vi "Read_Sc.vi"(3 "error in (no error)":errorcluster, 4 "timeout ms (10000)":i32=10000, 5 "connection ID":refnum<k5>) -> (0 "error out":errorcluster, 1 "data out":string, 2 "connection ID out":refnum<k5>)   [LabVIEW 2015]
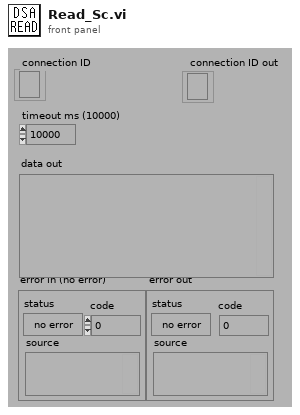
[diagram p1: front panel]
types:
  T1 = enum16{"Standard", "Buffered", "CRLF", "Immediate"}
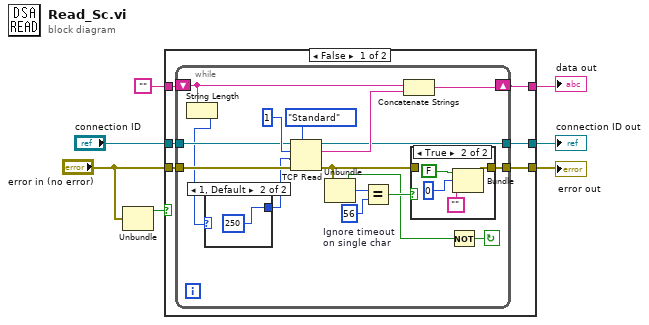
[diagram p0: block diagram]
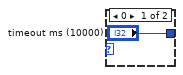
[diagram p2: hidden frame]
diagram:
  n1 = Unbundle("error in (no error)") -> ("status"=w6:bool)  [unwired: 2 out]
  n2 = case shown="False" w6 {
    tunnel: [w13 w39] -> w7
    tunnel: "error in (no error)" -> [w12 w40]
    tunnel: "connection ID" -> [w11 w38]
    tunnel: [w10 w40] -> w3
    tunnel: "" -> [w9 w39]
    tunnel: [w8 w38] -> w1
    frame False {
      n3 = while {
        tunnel: [w20] -> w8
        tunnel: [w21] -> w10
        tunnel: w11 -> [w22]
        tunnel: w12 -> [w23]
        shift-left: w9 -> [w14]
        shift-right: [w25] -> w13
        stop <- w18 continue-if-true
        w29 = 56  # Ignore timeout on single char
        n4 = String Length(string=w14) -> (length=w15:i32)
        n5 = case shown="1, Default" w15 {
          tunnel: ["timeout ms (10000)" 250] -> w16
          frame 0 {
          }
          frame 1, Default {
          }
        }
        n6 = TCP Read(connection ID=w22, bytes to read=1, error in (no error)=w23, 7:T1."Standard" ("mode (standard)"), 9:w16) -> (connection ID out=w20:refnum<k5>, data out=w24:string, error out=w30:errorcluster)
        n7 = Unbundle(w30) -> ("status"=w19:bool, "code"=w28:i32)  [unwired: 1 out]
        n8 = Equal?(x=w28, y=w29) -> (x = y?=w27:bool)
        n9 = Concatenate Strings(w14, w24) -> (w25:string)
        n10 = case shown="True" w27 {
          tunnel: [w33 w34] -> w21
          tunnel: w30 -> [w33 _]
          frame False {
          }
          frame True {
            n11 = Bundle(FALSE, 0, "") -> (w34:errorcluster)  [unwired: 1 in]
          }
        }
        n12 = Not(x=w19) -> (.not. x?=w18:bool)
      }
    }
    frame True {
    }
  }
  "connection ID out" <- w1
  "error out" <- w3
  "data out" <- w7
